vi "TelemetryServer_Global.vi"() -> ()   [LabVIEW 2009]
panel:
  in  "TelemetryWaveform":waveform(dbl)={"t0"=timestamp(0 s since 1904-01-01), "dt"=0.0, "Y"=[]} caption="TelemetryData"
  out "TelemetryServerPacket event":refnum<user-event>
  in  "TelemetryServerPacket":T1
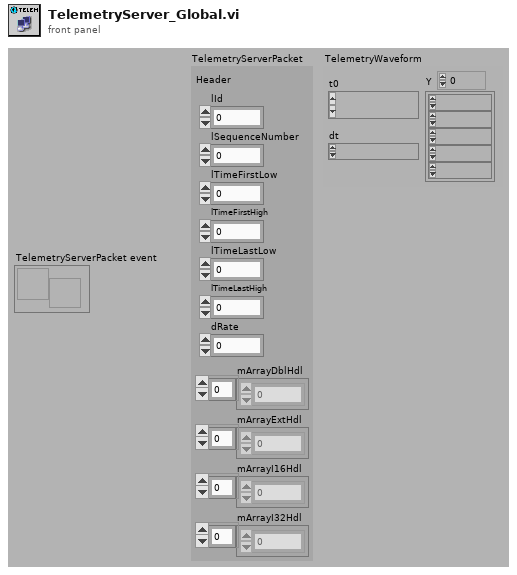
[diagram p1: front panel]
types:
  T1 = cluster{"Header":cluster{"lId":u32, "lSequenceNumber":u32, "lTimeFirstLow":u32, "lTimeFirstHigh":u32, "lTimeLastLow":u32, "lTimeLastHigh":u32, "dRate":dbl}, "mArrayDblHdl":dbl[], "mArrayExtHdl":ext[], "mArrayI16Hdl":i16[], "mArrayI32Hdl":i32[]}
diagram:
